vi "ultrasonic basic program.vi"   [LabVIEW 2012, in "sumobot 18.lvrbt"]
uses:
  sumobot 18.lvrbt
  <vilib>/NXT/Block Support/NXT_InputPort.ctl
  <vilib>/NXT/Block Support/NXT_OutputPort.ctl
  <vilib>/NXT/Dual Mode Library/Waits/Wait_Num.vi
  <vilib>/NXT/Dual Mode Library/Sensors/Sonar_cm.vi
  <vilib>/NXT/NXTIO Xnodes/NXTIONodeSubVIs/NXTMoveMotors.vi
  <vilib>/NXT/Subs/LVHSConnector.ctl
  <vilib>/NXT/NXTIO Xnodes/AddressXNode/NXTIOAddress.xnode
  <vilib>/NXT/NXTIO Xnodes/NXTIOXNode/NXTIO.xnode
  <vilib>/NXT/LegoClasses/BrickReference/BrickReference.lvclass
types:
  T1 = typedef "NXT_OutputPort.ctl" = u8
  T2 = cluster{"Output Port":T1, "Output Port 2":T1, "Output Port 3":T1}
  T3 = typedef "NXT_InputPort.ctl" = u32
  T4 = typedef "LVHSConnector.ctl" = refnum<class "BrickReference.lvclass">
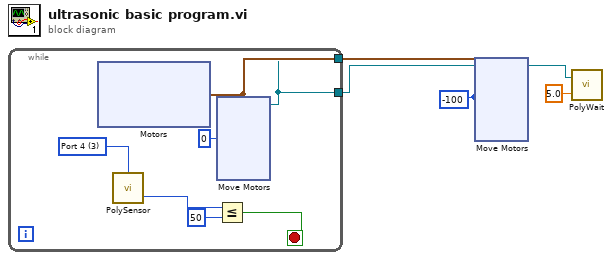
[diagram p0: block diagram]
diagram:
  w5 = i8 -100 ("Power/Speed 1")
  n1 = while {
    tunnel: [w7] -> w4
    tunnel: [w6] -> _
    tunnel: [w6] -> w1
    stop <- w8 stop-if-true
    w11 = T3 3 items=["Port 1", "Port 2", "Port 3", "Port 4"] ("Port (Port 4)")
    w12 = i8 0 ("Power/Speed 1")
    n2 = xnode "Motors"() -> ("Motor"=w7:cluster{"Port":T1, "Port":T1, "Port":T1})
    n3 = call-poly <vilib>:"PolySensor.vi"("Port (Port 4)"=w11) -> ("Distance (cm)"=w10:i16)  [unwired: 2 in, 1 out]
    n4 = xnode "Move Motors"("Power/Speed 3"=w12, "Power/Speed 2"=w12, "Power/Speed 1"=w12, "Motors"=w7) -> ("NXT/EV3"=w6:T4)  [unwired: 1 in]
    n5 = Less Or Equal?(x=w10, y=i16 50) -> (x <= y?=w8:bool)
  }
  n6 = xnode "Move Motors"("Power/Speed 3"=w5, "Power/Speed 1"=w5, "Motors"=w4, "NXT/EV3"=w1) -> ("NXT/EV3"=w3:T4)  [unwired: 1 in]
  n7 = call-poly <vilib>:"PolyWait.vi"("Time (1 sec)"=sgl 5.0, "NXT/EV3"=w3) -> ()  [unwired: 2 in, 1 out]
